vi "SendRoutedMessage.vi"(7 "listener process":string, 8 "error in (no error)":errorcluster, 9 "message value":variant, 10 "message name":string, 11 "Qbus in":refnum<class "Qbus.lvclass">) -> (0 "error in (no error)":errorcluster, 3 "Qbus out":refnum<class "Qbus.lvclass">)   [LabVIEW 2017, in "Qbus.lvclass"]
doc: "Sends a Qbus message to a specific \nprocess."
uses:
  <vilib>/addons/Qbus/Qbus.lvclass
  <vilib>/addons/Qbus/Qbus.lvclass/Qbus.ctl
  <vilib>/addons/Qbus/controls/message.ctl
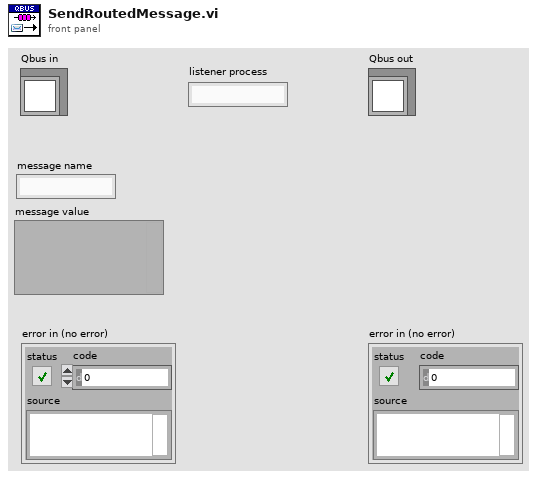
[diagram p1: front panel]
types:
  T1 = typedef "Qbus.lvclass/message.ctl" = cluster{"MsgName":string, "MsgValue":variant}
  T2 = typedef "Qbus.lvclass/data.ctl" = cluster{"Queues":variant, "Subscriptions":variant, "MasterQ":string}
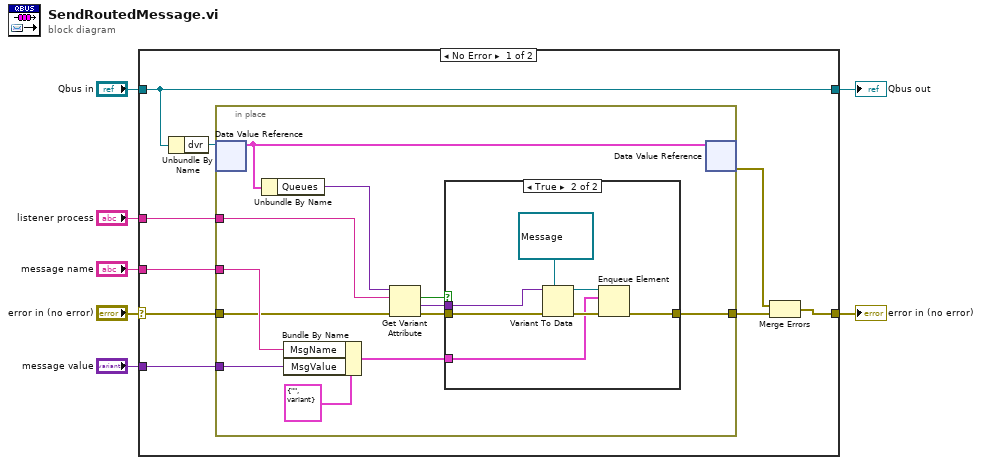
[diagram p0: block diagram]
diagram:
  n1 = case shown="No Error" "error in (no error)" {
    selector: "error in (no error)" -> [w13 w38]
    tunnel: [w12 w38] -> w6
    tunnel: [w16 w37] -> w4
    tunnel: "Qbus in" -> [w16 w37]
    tunnel: "message name" -> [w10 _]
    tunnel: "message value" -> [w9 _]
    tunnel: "listener process" -> [w8 _]
    frame No Error {
      n2 = Unbundle By Name(w16) -> ("dvr"=w15:refnum<data-value>)
      n3 = in-place {
        in-place-border: w13 -> [w22]
        in-place-border: [w27] -> w11
        in-place-border: w10 -> [w25]
        in-place-border: w9 -> [w24]
        in-place-border: w8 -> [w21]
        n4 = in-place-dvr #1(w15) -> (w28:T2)  [unwired: 1 out]
        n5 = Unbundle By Name(w28) -> ("Queues"=w20:variant)
        n6 = Bundle By Name(cluster=T1 {"MsgName"="", "MsgValue"=variant} ("Message"), "MsgName"=w25, "MsgValue"=w24) -> (w23:T1)
        n7 = Get Variant Attribute(Variant=w20, name=w21, error in=w22) -> (found=w18:bool, value=w17:variant, error out=w19:errorcluster)  [unwired: 1 in, 1 out]
        n8 = case shown="True" w18 {
          tunnel: w19 -> [w29 w30]
          tunnel: [w29 w34] -> w27
          tunnel: w23 -> [_ w32]
          tunnel: w17 -> [_ w31]
          frame False {
          }
          frame True {
            n9 = Variant To Data(error in=w30, type=refnum<queue> refnum ("queue out"), Variant=w31) -> (data=w33:refnum<queue>, error out=w35:errorcluster)
            n10 = Enqueue Element(queue=w33, element=w32, error in (no error)=w35) -> (error out=w34:errorcluster)  [unwired: 1 in, 2 out]
          }
        }
        n11 = in-place-dvr #1(w28) -> (w14:errorcluster)  [unwired: 1 out]
      }
      n12 = Merge Errors(w14, w11) -> (w12:errorcluster)
    }
    frame Error {
    }
  }
  "error in (no error)" <- w6
  "Qbus out" <- w4
